vi "testout.vi"() -> ()   [LabVIEW 2015]
uses:
  <vilib>/Platform/TimedLoop/XDataNode/timing_clust.ctl
  <vilib>/Platform/TimedLoop/XDataNode/nitl_modes.ctl
  <vilib>/Platform/TimedLoop/XDataNode/wakeup.ctl
  <vilib>/rvi/Emulation/niFpgaSctlEmulationGetInTimedLoop.vi
  <vilib>/rvi/Emulation/niFpgaEmulationReportErrorSimple.vi
  <vilib>/rvi/Emulation/niFpgaGetClockAttributes.vi
  <vilib>/rvi/Emulation/niFpgaCriticalErrorInLSC.vi
  <vilib>/rvi/eio/common/nirviEmuTemplateMethod_errors.vi
  <vilib>/Platform/TimedLoop/XDataNode/XDataNode.xnode
  <vilib>/eio/EIONode/EIONode.xnode
  <vilib>/Platform/TimedLoop/XDataNode/XDNodeRunTimeDep.lvlib
panel:
  out "IO Module\\AI 1":i16
  out "IO Module\\AI 0":i16
  in  "DIO 0":u8
  in  "DIO 1":u8
  in  "PFI 3":bool
  in  "PFI 2":bool
  in  "PFI 1":bool
  in  "PFI 0":bool
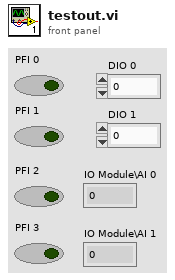
[diagram p1: front panel]
types:
  T1 = typedef "XDNodeRunTimeDep.lvlib/timing_clust.ctl" = cluster{"Expected End [f-1]":u64, "Actual End [f-1]":u64, "Finished Late? [f-1]":bool, "Expected End [i-1]":u64, "Actual End [i-1]":u64, "Finished Late? [i-1]":bool, "Expected Start [i]":u64, "Actual Start [i]":u64, "Expected Start [f]":u64, "Actual Start [f]":u64, "Source Name":string, "Structure Name":string, "Period":i64, "Deadline":i64, "Offset":i64, "Start":i64, "Priority":i32, "Timeout":i32, "Mode":T2, "Wakeup Reason":T3, "Error":errorcluster, "Source Type":string, "Secondary Source Type":string, "Global End Time":u64, "Global Start Time":u64, "Frame Duration":u64, "Iteration Duration":u64, "Assigned CPU":i32, "I/O Scan Engine Mode":u32}
  T2 = typedef "XDNodeRunTimeDep.lvlib/nitl_modes.ctl" = enum32{"No Change", "Process missed periods, maintain original phase", "Discard missed periods, maintain original phase", "Process missed periods, ignore original phase", "Discard missed periods, ignore original phase"}
  T3 = typedef "XDNodeRunTimeDep.lvlib/wakeup.ctl" = enum32{"Normal", "Aborted", "Asynchronous wakeup", "Timing source error", "Timed loop error", "Timeout"}
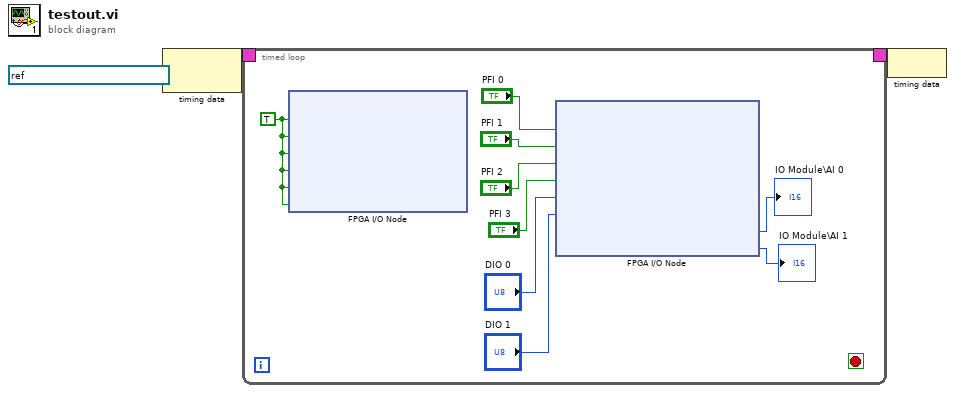
[diagram p0: block diagram]
diagram:
  n1 = node-c288(refnum<k21> "IO Module\\Sample Clock" ("Source Name")) -> (w3:T1)
  n2 = timed-loop {
    timing: w3 -> [_]
    timing-out: [_] -> w2
    stop <- _ stop-if-true
    w12 = TRUE ("IO Module\\PFI 0 WE")
    n3 = xnode "FPGA I/O Node"("IO Module\\PFI 0 WE"=w12, "IO Module\\PFI 1 WE"=w12, "IO Module\\PFI 2 WE"=w12, "IO Module\\PFI 3 WE"=w12, "IO Module\\DIO Port 0 WE"=w12, "IO Module\\DIO Port 1 WE"=w12) -> ()  [unwired: 6 in, 6 out]
    n4 = xnode "FPGA I/O Node"("IO Module\\PFI 0 Wr Data"="PFI 0", "IO Module\\PFI 1 Wr Data"="PFI 1", "IO Module\\PFI 2 Wr Data"="PFI 2", "IO Module\\PFI 3 Wr Data"="PFI 3", "IO Module\\DIO Port 0 Wr Data"="DIO 0", "IO Module\\DIO Port 1 Wr Data"="DIO 1") -> ("IO Module\\AI 0"=→"IO Module\\AI 0":u16, "IO Module\\AI 1"=→"IO Module\\AI 1":u16)  [unwired: 8 in, 8 out]
  }
  n5 = node-c288(w2) -> ()
